vi "Parse Logging Properties.vi"(11 "String":string) -> (3 "Logging properties":T1)   [LabVIEW 2015, in "NI_Azure_Queue.lvlib"]
uses:
  NI_Azure_Queue.lvlib
  Logging.ctl
  Retention Policy.ctl
  XML Parsing/NI_Azure_XML Parsing.lvlib
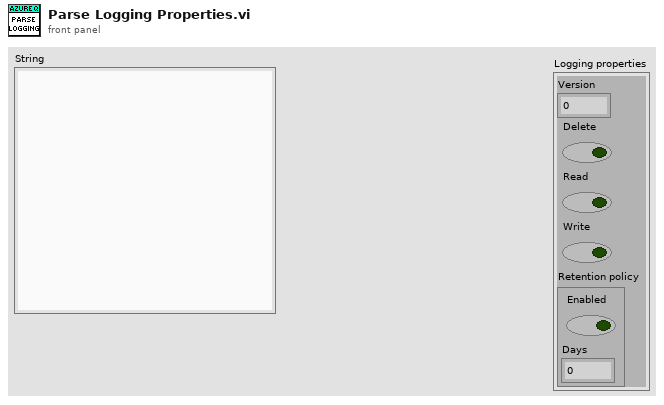
[diagram p1: front panel]
types:
  T1 = typedef "NI_Azure_Queue.lvlib/Logging.ctl" = cluster{"Version":dbl, "Delete":bool, "Read":bool, "Write":bool, "Retention policy":T2}
  T2 = typedef "NI_Azure_Queue.lvlib/Retention Policy.ctl" = cluster{"Enabled":bool, "Days":u32}
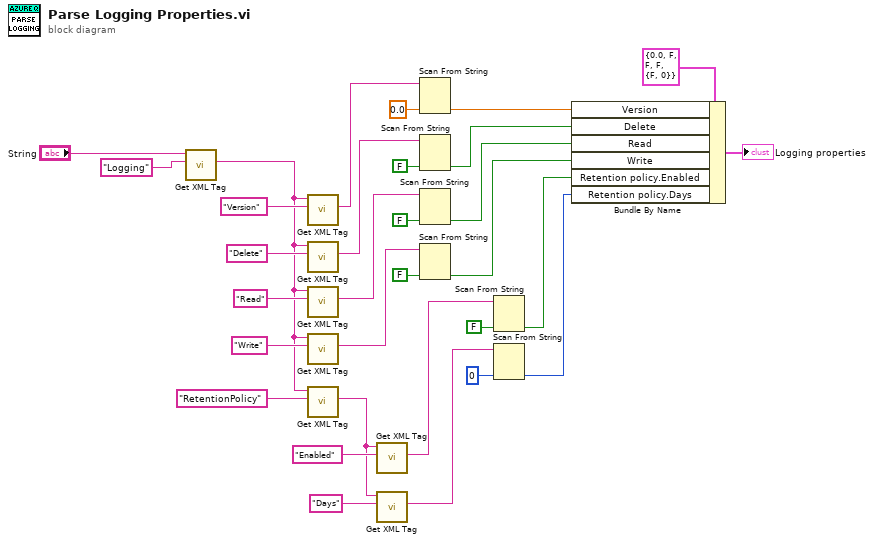
[diagram p0: block diagram]
diagram:
  n1 = call "Get XML Tag.vi"("Tag name"="Logging", "XML String in"="String") -> ("Tag value"=w22:string)  [unwired: 5 in, 4 out]
  n2 = call "Get XML Tag.vi"("Tag name"="Version", "XML String in"=w22) -> ("Tag value"=w15:string)  [unwired: 5 in, 4 out]
  n3 = call "Get XML Tag.vi"("Tag name"="Delete", "XML String in"=w22) -> ("Tag value"=w18:string)  [unwired: 5 in, 4 out]
  n4 = call "Get XML Tag.vi"("Tag name"="Read", "XML String in"=w22) -> ("Tag value"=w11:string)  [unwired: 5 in, 4 out]
  n5 = call "Get XML Tag.vi"("Tag name"="Write", "XML String in"=w22) -> ("Tag value"=w8:string)  [unwired: 5 in, 4 out]
  n6 = call "Get XML Tag.vi"("Tag name"="RetentionPolicy", "XML String in"=w22) -> ("Tag value"=w19:string)  [unwired: 5 in, 4 out]
  n7 = call "Get XML Tag.vi"("Tag name"="Enabled", "XML String in"=w19) -> ("Tag value"=w5:string)  [unwired: 5 in, 4 out]
  n8 = call "Get XML Tag.vi"("Tag name"="Days", "XML String in"=w19) -> ("Tag value"=w1:string)  [unwired: 5 in, 4 out]
  n9 = Scan From String(input string=w15, default 1=0.0 ("Version")) -> (output 1=w13:dbl)  [unwired: 3 in, 3 out]
  n10 = Scan From String(input string=w18, default 1=FALSE) -> (output 1=w16:bool)  [unwired: 3 in, 3 out]
  n11 = Scan From String(input string=w11, default 1=FALSE) -> (output 1=w10:bool)  [unwired: 3 in, 3 out]
  n12 = Scan From String(input string=w8, default 1=FALSE) -> (output 1=w7:bool)  [unwired: 3 in, 3 out]
  n13 = Scan From String(input string=w5, default 1=FALSE) -> (output 1=w4:bool)  [unwired: 3 in, 3 out]
  n14 = Scan From String(input string=w1, default 1=u32 0 ("Retention policy.Days")) -> (output 1=w2:u32)  [unwired: 3 in, 3 out]
  n15 = Bundle By Name(cluster=T1 {"Version"=0.0, "Delete"=FALSE, "Read"=FALSE, "Write"=FALSE, "Retention policy"={"Enabled"=FALSE, "Days"=0}} ("Logging properties"), "Version"=w13, "Delete"=w16, "Read"=w10, "Write"=w7, "Retention policy.Enabled"=w4, "Retention policy.Days"=w2) -> (→"Logging properties":T1)
